vi "example_llm_anthropic_unit_test_1.vi"() -> ()   [LabVIEW 2020]
uses:
  src/models/message_text/message_text.lvclass
  D:/Personal/LabVIEW LLMs/src/models/abstract_message_base/abstract_message_base.lvclass
  src/models/llm_anthropic_chatmodels/llm_anthropic_chatmodels.lvclass
  D:/Personal/LabVIEW LLMs/src/models/abstract_llm_base/abstract_llm_base.lvclass
  src/models/message_text/message.ctl
panel:
  in  "model_name":string(combo)="claude-3-5-sonnet-20240620"
  in  "temperature":dbl=1.0
  in  "Messages":cluster{"role":string, "text":string}[](array[cluster])=[{"role"="system", "text"="Act as a math teacher and guide the student in solving the problem. You should not solve the problem. Always answer in single line."}, {"role"="user", "text"="What is x in the equation 2x + 3 = 5  ?"}]
  out "error out":errorcluster
  out "anthropic_key":string
  # "1. Ensure you assign the Anthropic Key to environmental variables so it is away from the code and easy to use the examples in future.\n\n2. Use the \"Set_Env_Var.vi\" from examples/utils folder to set the key \"labview_llm_anthropic_key\"."
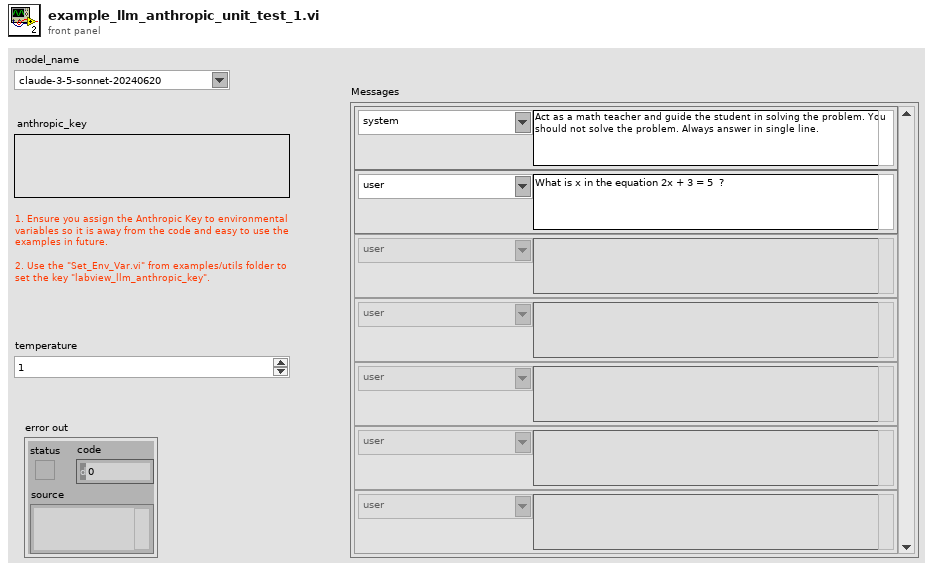
[diagram p1: front panel]
types:
  T1 = typedef "message_text.lvclass/message.ctl" = cluster{"role":string, "content":string[]}
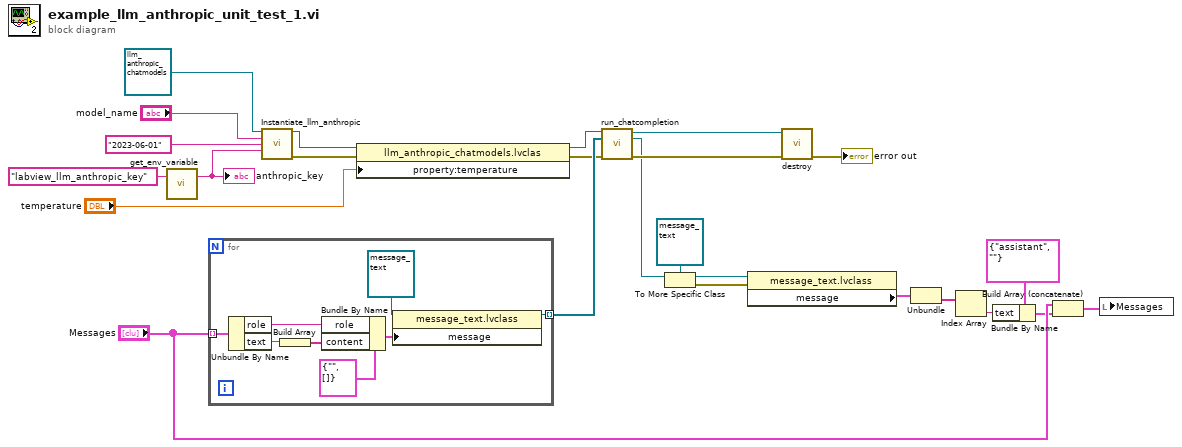
[diagram p0: block diagram]
diagram:
  n1 = call "get_env_variable.vi"("Environment Variable Name"="labview_llm_anthropic_key") -> ("Value"=w1:string)  [unwired: 1 in, 1 out]
  "anthropic_key" <- w1
  n2 = for {
    tunnel: "Messages" -> [w31] mode=indexing
    tunnel: [w32] -> w21 mode=indexing
    n3 = Unbundle By Name(w31) -> ("role"=w29:string, "text"=w27:string)
    n4 = Build Array(w27) -> (w26:string[])
    n5 = Bundle By Name(cluster=T1 {"role"="", "content"=[]} ("message"), "role"=w29, "content"=w26) -> (w28:T1)
    n6 = property class="message_text.lvclass"(reference=refnum<class "message_text.lvclass"> refnum ("message_text.lvclass"), "message"=w28) -> (reference out=w32:refnum<class "message_text.lvclass">)  [unwired: 1 in, 1 out]
  }
  n7 = call "Instantiate_llm_anthropic.vi"("llm_anthropic_chatmodels in"=refnum<class "llm_anthropic_chatmodels.lvclass"> refnum ("llm_anthropic_chatmodels.lvclass"), "model_name"="model_name", "anthropic_version"="2023-06-01", "anthropic_key"=w1) -> ("llm_anthropic_chatmodels out"=w5:refnum<class "llm_anthropic_chatmodels.lvclass">, "error out"=w4:errorcluster)  [unwired: 10 in]
  n8 = property class="llm_anthropic_chatmodels.lvclas"(reference=w5, error in=w4, "property:temperature"="temperature") -> (reference out=w18:refnum<class "llm_anthropic_chatmodels.lvclass">, error out=w17:errorcluster)
  n9 = call-dynamic "run_chatcompletion.vi"("llm_anthropic_chatmodels in"=w18, "Messages"=w21, "error in (no error)"=w17) -> ("llm_anthropic_chatmodels out"=w25:refnum<class "llm_anthropic_chatmodels.lvclass">, "Response"=w8:refnum<class "abstract_message_base.lvclass">, "error out"=w24:errorcluster)  [unwired: 10 in]
  n10 = To More Specific Class(target class=refnum<class "message_text.lvclass"> refnum ("message_text.lvclass"), reference=w8) -> (specific class reference=w9:refnum<class "message_text.lvclass">, error out=w11:errorcluster)  [unwired: 1 in]
  n11 = property class="message_text.lvclass"(reference=w9, error in=w11) -> ("message"=w14:T1)  [unwired: 2 out]
  n12 = call-dynamic "destroy.vi"("error in (no error)"=w24, "abstract_llm_base in"=w25) -> ("error out"=→"error out":errorcluster)  [unwired: 8 in, 1 out]
  n13 = Unbundle(w14) -> ("content"=w13:string[])  [unwired: 1 out]
  n14 = Index Array(array=w13) -> (element=w12:string)  [unwired: 1 in]
  n15 = Bundle By Name(cluster=cluster{"role":string, "text":string} {"role"="assistant", "text"=""} ("message"), "text"=w12) -> (w7:cluster{"role":string, "text":string})
  n16 = Build Array (concatenate)("Messages", w7) -> (w19:cluster{"role":string, "text":string}[])
  n17 = local write "Messages"(w19) -> ()
